vi "Get U16.vi"(8 "error in (no error)":errorcluster, 9 "Data Type (default value)":u16, 10 "Offset":i32, 11 "JSON":string) -> (0 "error out":errorcluster, 1 "Number":u16, 2 "Offset past match":i32)   [LabVIEW 2024, in "JSONtext.lvlib"]
uses:
  JSONtext.lvlib
  String Subset.vi
  Advance past Number.vi
  Format Error.vi
  Parsing Error in converting to LabVIEW type.vi
  Error Cluster From Error Code.vi
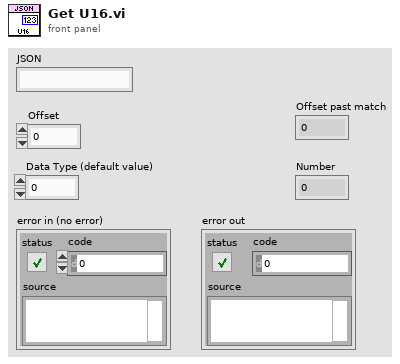
[diagram p1: front panel]
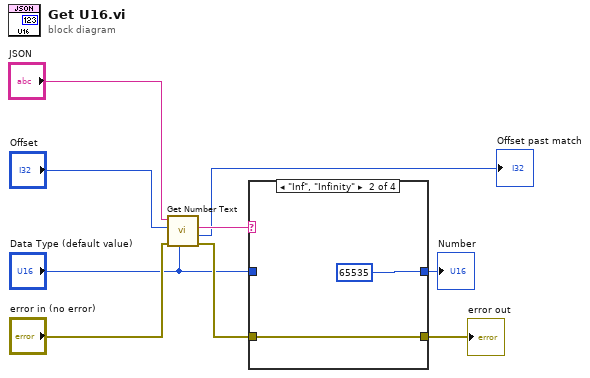
[diagram p0: block diagram]
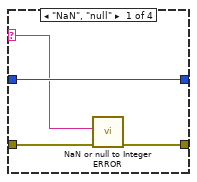
[diagram p2: hidden frame]
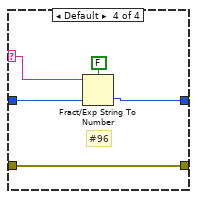
[diagram p4: hidden frame]
diagram:
  n1 = call "Get Number Text.vi"("LV Type"="Data Type (default value)", "error in (no error)"="error in (no error)", "Offset"="Offset", "JSON"="JSON") -> ("error out"=w6:errorcluster, "Offset past match"=→"Offset past match":i32, "Number Text"=w4:string)  [unwired: 4 in, 1 out]
  n2 = case shown="\"Inf\", \"Infinity\"" w4 {
    selector: w4 -> [w10 _ _ w17]
    tunnel: [w13 u16 65535 ("default value 1") _ w19] -> w3
    tunnel: w6 -> [w12 w14 w16 w18]
    tunnel: [w11 w14 w16 w18] -> w5
    tunnel: "Data Type (default value)" -> [w13 _ _ w20]
    frame "NaN", "null" {
      n3 = call "NaN or null to Integer ERROR.vi"("error in (no error)"=w12, "JSON NaN or null"=w10) -> ("error out"=w11:errorcluster)  [unwired: 9 in]
    }
    frame "Inf", "Infinity" {
    }
    frame "-Inf", "-Infinity" {
      # "2022-5-19 change to zero\nrather than default value,\nto be consistant with\nlarge negative numbers"
    }
    frame Default {
      # "#96"
      n4 = Fract/Exp String To Number(use system decimal point (T)=FALSE, string=w17, default (0 dbl)=w20) -> (number=w19:u16)  [unwired: 1 in, 1 out]
    }
  }
  "error out" <- w5
  "Number" <- w3
